vi "Diode-Test2-Array.vi"() -> ()   [LabVIEW 2020]
uses:
  Diode-SCPI-Driver/Diode-Keyword.ctl
panel:
  in  "Stop":bool
  out "Waveform Graph":u16[][](graph)=[[6664, 5392, 4415, 3740, 3338, 2832, 2456, 2200, 1952, 1855, 1920, 1848, 1808, 1698, 1703, 1756, 1820, 1796, 1664, 1584, 1495, 1648, 1584, 1536, 1416, 1424, 1432, 1468, 1588, 1552, 1480, 1488, 1536, 1388, 1432, 1468, 1592, 1576, 1465, 1590, 1580, 1584, 1488, 1536, 1384, 1408, 1343, 1467, 1594, 1584, 1552, 1456, 1492, 1544, 1464, 1536, 1416, 1418, 1469, 1576, 1488, 1540, 1424, 1462, 1542, 1538, 1420, 1470, 1597, 1599, 1672, 1591, 1599, 1696, 1599, 1680, 1664, 1544, 1468, 1557, 1521, 1550, 1560, 1468, 1595, 1592, 1568, 1458, 1577, 1510, 1595, 1627, 1664, 1569, 1432, 1498, 1592, 1570, 1536, 1386, 1407, 1570, 1536, 1410, 1408, 1408, 1340, 1424, 1425, 1416, 1409, 1408, 1343, 1462, 1599, 1664, 1577, 1484, 1564, 1534, 1720, 1744, 1727, 1855, 1855, 1936, 1820, 1836, 1776, 1808, 1688, 1681, 1599, 1705, 1672, 1596, 1599, 1680, 1664, 1550, 1570, 1468, 1597, 1592, 1554, 1518, 1664, 1558, 1587, 1564, 1552, 1460, 1552, 1460, 1536, 1424, 1416, 1424, 1414, 1471, 1664, 1561, 1496, 1593, 1560, 1496, 1568, 1464, 1558, 1536, 1430, 1492, 1590, 1564, 1568, 1432, 1488, 1544, 1457, 1470, 1632, 1537, 1424, 1424, 1424, 1456, 1458, 1588, 1536, 1426, 1456, 1471, 1664, 1560, 1492, 1553, 1458, 1577, 1470, 1656, 1672, 1592, 1578, 1548, 1536, 1343, 1456, 1498, 1594, 1598, 1664, 1578, 1562, 1567, 1599, 1668, 1595, 1632, 1536, 1408, 1342, 1490, 1552, 1456, 1490, 1576, 1470, 1664, 1584, 1504, 1514, 1599, 1668, 1599, 1680, 1598, 1680, 1599, 1688, 1688, 1688, 1680, 1632, 1560, 1496, 1546, 1536, 1408, 1342, 1470, 1632, 1552, 1456, 1494, 1599, 1599, 1680, 1664, 1577, 1496, 1584, 1536, 1343, 1492, 1560, 1494, 1592, 1579, 1552, 1454, 1560, 1536, 1343, 1492, 1560, 1504, 1514, 1593, 1570, 1552, 1432, 1468, 1580, 1552, 1454, 1560, 1538, 1436, 1552, 1424, 1443, 1456, 1536, 1342, 1491, 1552, 1447, 1520, 1598, 1599, 1698, 1688, 1690, 1720, 1776, 1724, 1794, 1672, 1680, 1598, 1670, 1672, 1666, 1592, 1595, 1580, 1584, 1468, 1594, 1598, 1664, 1566, 1584, 1538, 1457, 1492, 1584, 1497, 1584, 1496, 1598, 1664, 1560, 1556, 1468, 1592, 1560, 1536, 1408, 1336, 1380, 1333, 1392, 1343, 1499, 1596, 1664, 1552, 1474, 1496, 1571, 1496, 1579, 1544, 1449, 1468, 1580, 1536, 1418, 1456, 1536, 1408, 1343, 1470, 1599, 1672, 1594, 1648, 1584, 1544, 1422, 1536, 1392, 1426, 1466, 1588, 1546, 1279, 1598, 1680, 1664, 1568, 1465, 1500, 1664, 1552, 1462, 1592, 1570, 1471, 1664, 1552, 1471, 1597, 1636, 1540, 1488, 1536, 1410, 1416, 1456, 1464, 1536, 1416, 1408, 1343, 1497, 1568, 1456, 1504, 1536, 1408, 1336, 1343, 1470, 1599, 1664, 1584, 1439, 1599, 1672, 1599, 1670, 1686, 1727, 1851, 1822, 1853, 1842, 1792, 1664, 1554, 1552, 1436, 1552, 1464, 1544, 1424, 1433, 1470, 1596, 1599, 1680, 1664, 1560, 1491, 1580, 1560, 1468, 1599, 1664, 1578, 1518, 1696, 1596, 1621, 1576, 1538, 1432, 1536, 1340, 1464, 1544, 1440, 1479, 1577, 1470, 1664, 1588, 1569, 1448, 1464, 1568, 1420, 1475, 1496, 1634, 1538, 1490, 1548, 1536, 1343, 1488, 1536, 1410, 1408, 1408, 1340, 1416, 1416, 1433, 1468, 1587, 1558, 1576, 1490, 1592, 1556, 1467, 1571, 1536, 1424, 1408, 1408, 1311, 1442, 1468, 1570, 1536, 1416, 1412, 1441, 1416, 1432, 1439, 1596, 1598, 1648, 1599, 1672, 1632, 1524, 1706, 1678, 1748, 1724, 1814, 1749, 1792, 1590, 1664, 1560, 1536, 1408, 1394, 1424, 1456, 1460, 1536, 1408, 1343, 1463, 1567, 1598, 1672, 1599, 1680, 1598, 1680, 1599, 1672, 1599, 1696, 1598, 1681, 1664, 1576, 1508, 1552, 1464, 1536, 1408, 1340, 1430, 1470, 1667, 1599, 1700, 1664, 1589, 1552, 1459, 1520, 1582, 1584, 1550, 1500, 1664, 1536, 1424, 1428, 1536, 1340, 1408, 1343, 1459, 1538, 1461, 1516, 1599, 1680, 1598, 1676, 1712, 1684, 1692, 1736, 1705, 1676, 1696, 1664, 1554, 1506, 1598, 1622, 1680, 1599, 1680, 1596, 1599, 1672, 1590, 1596, 1599, 1672, 1664, 1569, 1464, 1536, 1416, 1408, 1393, 1408, 1343, 1464, 1560, 1470, 1665, 1576, 1536, 1408, 1337, 1343, 1432, 1507, 1552, 1475, 1471, 1636, 1596, 1599, 1664, 1590, 1594, 1618, 1576, 1554, 1464, 1554, 1492, 1568, 1468, 1568, 1450, 1552, 1428, 1471, 1664, 1559, 1548, 1471, 1664, 1560, 1536, 1343, 1536, 1341, 1425, 1424, 1442, 1436, 1550, 1520, 1590, 1594, 1664, 1552, 1470, 1598, 1684, 1664, 1592, 1536, 1426, 1464, 1538, 1436, 1568, 1420, 1490, 1548, 1506, 1552, 1463, 1568, 1470, 1599, 1664, 1574, 1568, 1536, 1408, 1343, 1466, 1566, 1599, 1664, 1585, 1512, 1584, 1508, 1568, 1465, 1536, 1424, 1412, 1441, 1408, 1343, 1458, 1552, 1450, 1536, 1416, 1424, 1410, 1448, 1468, 1584, 1510, 1597, 1599, 1648, 1594, 1599, 1672, 1599, 1670, 1696, 1664, 1560, 1506, 1570, 1495, 1599, 1680, 1664, 1542, 1536, 1392, 1408, 1408, 1342, 1471, 1598, 1676, 1670, 1664, 1596, 1584, 1538, 1424, 1476, 1468, 1596, 1564, 1566, 1576, 1536, 1343, 1494, 1598, 1682, 1672, 1631, 1688, 1680, 1597, 1634, 1592, 1555, 1536, 1394, 1432, 1494, 1582, 1664, 1536, 1450, 1492, 1574, 1503, 1684, 1694, 1812, 1704, 1715, 1727, 1851, 1840, 1760, 1692, 1739, 1727, 1854, 1896, 1840, 1758, 1855, 1886, 1953, 1852, 1855, 1900, 1855, 1823, 1855, 1920, 1840, 1726, 1848, 1798, 1753, 1663, 1816, 1727, 1840, 1776, 1751, 1840, 1808, 1698, 1692, 1738, 1725, 1824, 1668, 1664, 1548, 1536, 1343, 1470, 1624, 1599, 1664, 1584, 1536, 1408, 1342, 1459, 1536, 1408, 1343, 1470, 1598, 1680, 1664, 1566, 1598, 1672, 1590, 1599, 1664, 1586, 1552, 1464, 1548, 1465, 1574, 1552, 1455, 1564, 1568, 1432, 1536, 1332, 1408, 1326, 1432, 1454, 1596, 1576, 1538, 1432, 1470, 1630, 1680, 1640, 1594, 1588, 1598, 1664, 1584, 1536, 1401, 1444, 1456, 1504, 1488, 1542, 1460, 1560, 1470, 1666, 1598, 1680, 1628, 1599, 1674, 1696, 1599, 1664, 1586, 1584, 1503, 1689, 1684, 1672, 1634, 1592, 1570, 1488, 1552, 1436, 1538, 1424, 1440, 1432, 1471, 1664, 1584, 1500, 1595, 1594, 1599, 1700, 1664, 1578, 1560, 1536, 1342, 1488, 1486, 1624, 1566, 1599, 1599, 1694, 1723, 1842, 1792, 1599, 1688, 1704, 1668, 1639, 1664, 1584, 1504, 1536, 1408, 1342, 1460, 1592, 1576, 1471, 1664, 1565, 1544, 1440, 1456, 1457, 1520, 1552, 1470, 2860, 2489, 2304, 1855, 1928, 1850, 1855, 1952, 1846, 1872, 574, 831, 1036, 1059, 1048, 1074, 1087, 1210, 1343, 1440, 1440, 1460, 1552, 1440, 1456]]
  out "array":u16[][](array[numeric])=[[6664, 5392, 4415, 3740, 3338, 2832, 2456, 2200, 1952, 1855, 1920, 1848, 1808, 1698, 1703, 1756, 1820, 1796, 1664, 1584, 1495, 1648, 1584, 1536, 1416, 1424, 1432, 1468, 1588, 1552, 1480, 1488, 1536, 1388, 1432, 1468, 1592, 1576, 1465, 1590, 1580, 1584, 1488, 1536, 1384, 1408, 1343, 1467, 1594, 1584, 1552, 1456, 1492, 1544, 1464, 1536, 1416, 1418, 1469, 1576, 1488, 1540, 1424, 1462, 1542, 1538, 1420, 1470, 1597, 1599, 1672, 1591, 1599, 1696, 1599, 1680, 1664, 1544, 1468, 1557, 1521, 1550, 1560, 1468, 1595, 1592, 1568, 1458, 1577, 1510, 1595, 1627, 1664, 1569, 1432, 1498, 1592, 1570, 1536, 1386, 1407, 1570, 1536, 1410, 1408, 1408, 1340, 1424, 1425, 1416, 1409, 1408, 1343, 1462, 1599, 1664, 1577, 1484, 1564, 1534, 1720, 1744, 1727, 1855, 1855, 1936, 1820, 1836, 1776, 1808, 1688, 1681, 1599, 1705, 1672, 1596, 1599, 1680, 1664, 1550, 1570, 1468, 1597, 1592, 1554, 1518, 1664, 1558, 1587, 1564, 1552, 1460, 1552, 1460, 1536, 1424, 1416, 1424, 1414, 1471, 1664, 1561, 1496, 1593, 1560, 1496, 1568, 1464, 1558, 1536, 1430, 1492, 1590, 1564, 1568, 1432, 1488, 1544, 1457, 1470, 1632, 1537, 1424, 1424, 1424, 1456, 1458, 1588, 1536, 1426, 1456, 1471, 1664, 1560, 1492, 1553, 1458, 1577, 1470, 1656, 1672, 1592, 1578, 1548, 1536, 1343, 1456, 1498, 1594, 1598, 1664, 1578, 1562, 1567, 1599, 1668, 1595, 1632, 1536, 1408, 1342, 1490, 1552, 1456, 1490, 1576, 1470, 1664, 1584, 1504, 1514, 1599, 1668, 1599, 1680, 1598, 1680, 1599, 1688, 1688, 1688, 1680, 1632, 1560, 1496, 1546, 1536, 1408, 1342, 1470, 1632, 1552, 1456, 1494, 1599, 1599, 1680, 1664, 1577, 1496, 1584, 1536, 1343, 1492, 1560, 1494, 1592, 1579, 1552, 1454, 1560, 1536, 1343, 1492, 1560, 1504, 1514, 1593, 1570, 1552, 1432, 1468, 1580, 1552, 1454, 1560, 1538, 1436, 1552, 1424, 1443, 1456, 1536, 1342, 1491, 1552, 1447, 1520, 1598, 1599, 1698, 1688, 1690, 1720, 1776, 1724, 1794, 1672, 1680, 1598, 1670, 1672, 1666, 1592, 1595, 1580, 1584, 1468, 1594, 1598, 1664, 1566, 1584, 1538, 1457, 1492, 1584, 1497, 1584, 1496, 1598, 1664, 1560, 1556, 1468, 1592, 1560, 1536, 1408, 1336, 1380, 1333, 1392, 1343, 1499, 1596, 1664, 1552, 1474, 1496, 1571, 1496, 1579, 1544, 1449, 1468, 1580, 1536, 1418, 1456, 1536, 1408, 1343, 1470, 1599, 1672, 1594, 1648, 1584, 1544, 1422, 1536, 1392, 1426, 1466, 1588, 1546, 1279, 1598, 1680, 1664, 1568, 1465, 1500, 1664, 1552, 1462, 1592, 1570, 1471, 1664, 1552, 1471, 1597, 1636, 1540, 1488, 1536, 1410, 1416, 1456, 1464, 1536, 1416, 1408, 1343, 1497, 1568, 1456, 1504, 1536, 1408, 1336, 1343, 1470, 1599, 1664, 1584, 1439, 1599, 1672, 1599, 1670, 1686, 1727, 1851, 1822, 1853, 1842, 1792, 1664, 1554, 1552, 1436, 1552, 1464, 1544, 1424, 1433, 1470, 1596, 1599, 1680, 1664, 1560, 1491, 1580, 1560, 1468, 1599, 1664, 1578, 1518, 1696, 1596, 1621, 1576, 1538, 1432, 1536, 1340, 1464, 1544, 1440, 1479, 1577, 1470, 1664, 1588, 1569, 1448, 1464, 1568, 1420, 1475, 1496, 1634, 1538, 1490, 1548, 1536, 1343, 1488, 1536, 1410, 1408, 1408, 1340, 1416, 1416, 1433, 1468, 1587, 1558, 1576, 1490, 1592, 1556, 1467, 1571, 1536, 1424, 1408, 1408, 1311, 1442, 1468, 1570, 1536, 1416, 1412, 1441, 1416, 1432, 1439, 1596, 1598, 1648, 1599, 1672, 1632, 1524, 1706, 1678, 1748, 1724, 1814, 1749, 1792, 1590, 1664, 1560, 1536, 1408, 1394, 1424, 1456, 1460, 1536, 1408, 1343, 1463, 1567, 1598, 1672, 1599, 1680, 1598, 1680, 1599, 1672, 1599, 1696, 1598, 1681, 1664, 1576, 1508, 1552, 1464, 1536, 1408, 1340, 1430, 1470, 1667, 1599, 1700, 1664, 1589, 1552, 1459, 1520, 1582, 1584, 1550, 1500, 1664, 1536, 1424, 1428, 1536, 1340, 1408, 1343, 1459, 1538, 1461, 1516, 1599, 1680, 1598, 1676, 1712, 1684, 1692, 1736, 1705, 1676, 1696, 1664, 1554, 1506, 1598, 1622, 1680, 1599, 1680, 1596, 1599, 1672, 1590, 1596, 1599, 1672, 1664, 1569, 1464, 1536, 1416, 1408, 1393, 1408, 1343, 1464, 1560, 1470, 1665, 1576, 1536, 1408, 1337, 1343, 1432, 1507, 1552, 1475, 1471, 1636, 1596, 1599, 1664, 1590, 1594, 1618, 1576, 1554, 1464, 1554, 1492, 1568, 1468, 1568, 1450, 1552, 1428, 1471, 1664, 1559, 1548, 1471, 1664, 1560, 1536, 1343, 1536, 1341, 1425, 1424, 1442, 1436, 1550, 1520, 1590, 1594, 1664, 1552, 1470, 1598, 1684, 1664, 1592, 1536, 1426, 1464, 1538, 1436, 1568, 1420, 1490, 1548, 1506, 1552, 1463, 1568, 1470, 1599, 1664, 1574, 1568, 1536, 1408, 1343, 1466, 1566, 1599, 1664, 1585, 1512, 1584, 1508, 1568, 1465, 1536, 1424, 1412, 1441, 1408, 1343, 1458, 1552, 1450, 1536, 1416, 1424, 1410, 1448, 1468, 1584, 1510, 1597, 1599, 1648, 1594, 1599, 1672, 1599, 1670, 1696, 1664, 1560, 1506, 1570, 1495, 1599, 1680, 1664, 1542, 1536, 1392, 1408, 1408, 1342, 1471, 1598, 1676, 1670, 1664, 1596, 1584, 1538, 1424, 1476, 1468, 1596, 1564, 1566, 1576, 1536, 1343, 1494, 1598, 1682, 1672, 1631, 1688, 1680, 1597, 1634, 1592, 1555, 1536, 1394, 1432, 1494, 1582, 1664, 1536, 1450, 1492, 1574, 1503, 1684, 1694, 1812, 1704, 1715, 1727, 1851, 1840, 1760, 1692, 1739, 1727, 1854, 1896, 1840, 1758, 1855, 1886, 1953, 1852, 1855, 1900, 1855, 1823, 1855, 1920, 1840, 1726, 1848, 1798, 1753, 1663, 1816, 1727, 1840, 1776, 1751, 1840, 1808, 1698, 1692, 1738, 1725, 1824, 1668, 1664, 1548, 1536, 1343, 1470, 1624, 1599, 1664, 1584, 1536, 1408, 1342, 1459, 1536, 1408, 1343, 1470, 1598, 1680, 1664, 1566, 1598, 1672, 1590, 1599, 1664, 1586, 1552, 1464, 1548, 1465, 1574, 1552, 1455, 1564, 1568, 1432, 1536, 1332, 1408, 1326, 1432, 1454, 1596, 1576, 1538, 1432, 1470, 1630, 1680, 1640, 1594, 1588, 1598, 1664, 1584, 1536, 1401, 1444, 1456, 1504, 1488, 1542, 1460, 1560, 1470, 1666, 1598, 1680, 1628, 1599, 1674, 1696, 1599, 1664, 1586, 1584, 1503, 1689, 1684, 1672, 1634, 1592, 1570, 1488, 1552, 1436, 1538, 1424, 1440, 1432, 1471, 1664, 1584, 1500, 1595, 1594, 1599, 1700, 1664, 1578, 1560, 1536, 1342, 1488, 1486, 1624, 1566, 1599, 1599, 1694, 1723, 1842, 1792, 1599, 1688, 1704, 1668, 1639, 1664, 1584, 1504, 1536, 1408, 1342, 1460, 1592, 1576, 1471, 1664, 1565, 1544, 1440, 1456, 1457, 1520, 1552, 1470, 2860, 2489, 2304, 1855, 1928, 1850, 1855, 1952, 1846, 1872, 574, 831, 1036, 1059, 1048, 1074, 1087, 1210, 1343, 1440, 1440, 1460, 1552, 1440, 1456]]
  in  "max bytes to read (500)":i32=10000
  in  "Diode Keyword":T1={"Keyword"="DIOD:TRAC:YARR", "Gettable"=TRUE, "Settable"=FALSE, "Is Array"=FALSE, "Data Type"="string", "Description"="Identify the instrument."}
  out "Response":string="6664,5392,4415,3740,3338,2832,2456,2200,1952,1855,1920,1848,1808,1698,1703,1756,1820,1796,1664,1584,1495,1648,1584,1536,1416,1424,1432,1468,1588,1552,1480,1488,1536,1388,1432,1468,1592,1576,1465,1590,1580,1584,1488,1536,1384,1408,1343,1467,1594,1584,1552,1456,1492,1544,1464,1536,1416,1418,1469,1576,1488,1540,1424,1462,1542,1538,1420,1470,1597,1599,1672,1591,1599,1696,1599,1680,1664,1544,1468,1557,1521,1550,1560,1468,1595,1592,1568,1458,1577,1510,1595,1627,1664,1569,1432,1498,1592,1570,1536,1386,1407,1570,1536,1410,1408,1408,1340,1424,1425,1416,1409,1408,1343,1462,1599,1664,1577,1484,1564,1534,1720,1744,1727,1855,1855,1936,1820,1836,1776,1808,1688,1681,1599,1705,1672,1596,1599,1680,1664,1550,1570,1468,1597,1592,1554,1518,1664,1558,1587,1564,1552,1460,1552,1460,1536,1424,1416,1424,1414,1471,1664,1561,1496,1593,1560,1496,1568,1464,1558,1536,1430,1492,1590,1564,1568,1432,1488,1544,1457,1470,1632,1537,1424,1424,1424,1456,1458,1588,1536,1426,1456,1471,1664,1560,1492,1553,1458,1577,1470,1656,1672,1592,1578,1548,1536,1343,1456,1498,1594,1598,1664,1578,1562,1567,1599,1668,1595,1632,1536,1408,1342,1490,1552,1456,1490,1576,1470,1664,1584,1504,1514,1599,1668,1599,1680,1598,1680,1599,1688,1688,1688,1680,1632,1560,1496,1546,1536,1408,1342,1470,1632,1552,1456,1494,1599,1599,1680,1664,1577,1496,1584,1536,1343,1492,1560,1494,1592,1579,1552,1454,1560,1536,1343,1492,1560,1504,1514,1593,1570,1552,1432,1468,1580,1552,1454,1560,1538,1436,1552,1424,1443,1456,1536,1342,1491,1552,1447,1520,1598,1599,1698,1688,1690,1720,1776,1724,1794,1672,1680,1598,1670,1672,1666,1592,1595,1580,1584,1468,1594,1598,1664,1566,1584,1538,1457,1492,1584,1497,1584,1496,1598,1664,1560,1556,1468,1592,1560,1536,1408,1336,1380,1333,1392,1343,1499,1596,1664,1552,1474,1496,1571,1496,1579,1544,1449,1468,1580,1536,1418,1456,1536,1408,1343,1470,1599,1672,1594,1648,1584,1544,1422,1536,1392,1426,1466,1588,1546,1279,1598,1680,1664,1568,1465,1500,1664,1552,1462,1592,1570,1471,1664,1552,1471,1597,1636,1540,1488,1536,1410,1416,1456,1464,1536,1416,1408,1343,1497,1568,1456,1504,1536,1408,1336,1343,1470,1599,1664,1584,1439,1599,1672,1599,1670,1686,1727,1851,1822,1853,1842,1792,1664,1554,1552,1436,1552,1464,1544,1424,1433,1470,1596,1599,1680,1664,1560,1491,1580,1560,1468,1599,1664,1578,1518,1696,1596,1621,1576,1538,1432,1536,1340,1464,1544,1440,1479,1577,1470,1664,1588,1569,1448,1464,1568,1420,1475,1496,1634,1538,1490,1548,1536,1343,1488,1536,1410,1408,1408,1340,1416,1416,1433,1468,1587,1558,1576,1490,1592,1556,1467,1571,1536,1424,1408,1408,1311,1442,1468,1570,1536,1416,1412,1441,1416,1432,1439,1596,1598,1648,1599,1672,1632,1524,1706,1678,1748,1724,1814,1749,1792,1590,1664,1560,1536,1408,1394,1424,1456,1460,1536,1408,1343,1463,1567,1598,1672,1599,1680,1598,1680,1599,1672,1599,1696,1598,1681,1664,1576,1508,1552,1464,1536,1408,1340,1430,1470,1667,1599,1700,1664,1589,1552,1459,1520,1582,1584,1550,1500,1664,1536,1424,1428,1536,1340,1408,1343,1459,1538,1461,1516,1599,1680,1598,1676,1712,1684,1692,1736,1705,1676,1696,1664,1554,1506,1598,1622,1680,1599,1680,1596,1599,1672,1590,1596,1599,1672,1664,1569,1464,1536,1416,1408,1393,1408,1343,1464,1560,1470,1665,1576,1536,1408,1337,1343,1432,1507,1552,1475,1471,1636,1596,1599,1664,1590,1594,1618,1576,1554,1464,1554,1492,1568,1468,1568,1450,1552,1428,1471,1664,1559,1548,1471,1664,1560,1536,1343,1536,1341,1425,1424,1442,1436,1550,1520,1590,1594,1664,1552,1470,1598,1684,1664,1592,1536,1426,1464,1538,1436,1568,1420,1490,1548,1506,1552,1463,1568,1470,1599,1664,1574,1568,1536,1408,1343,1466,1566,1599,1664,1585,1512,1584,1508,1568,1465,1536,1424,1412,1441,1408,1343,1458,1552,1450,1536,1416,1424,1410,1448,1468,1584,1510,1597,1599,1648,1594,1599,1672,1599,1670,1696,1664,1560,1506,1570,1495,1599,1680,1664,1542,1536,1392,1408,1408,1342,1471,1598,1676,1670,1664,1596,1584,1538,1424,1476,1468,1596,1564,1566,1576,1536,1343,1494,1598,1682,1672,1631,1688,1680,1597,1634,1592,1555,1536,1394,1432,1494,1582,1664,1536,1450,1492,1574,1503,1684,1694,1812,1704,1715,1727,1851,1840,1760,1692,1739,1727,1854,1896,1840,1758,1855,1886,1953,1852,1855,1900,1855,1823,1855,1920,1840,1726,1848,1798,1753,1663,1816,1727,1840,1776,1751,1840,1808,1698,1692,1738,1725,1824,1668,1664,1548,1536,1343,1470,1624,1599,1664,1584,1536,1408,1342,1459,1536,1408,1343,1470,1598,1680,1664,1566,1598,1672,1590,1599,1664,1586,1552,1464,1548,1465,1574,1552,1455,1564,1568,1432,1536,1332,1408,1326,1432,1454,1596,1576,1538,1432,1470,1630,1680,1640,1594,1588,1598,1664,1584,1536,1401,1444,1456,1504,1488,1542,1460,1560,1470,1666,1598,1680,1628,1599,1674,1696,1599,1664,1586,1584,1503,1689,1684,1672,1634,1592,1570,1488,1552,1436,1538,1424,1440,1432,1471,1664,1584,1500,1595,1594,1599,1700,1664,1578,1560,1536,1342,1488,1486,1624,1566,1599,1599,1694,1723,1842,1792,1599,1688,1704,1668,1639,1664,1584,1504,1536,1408,1342,1460,1592,1576,1471,1664,1565,1544,1440,1456,1457,1520,1552,1470,2860,2489,2304,1855,1928,1850,1855,1952,1846,1872,574,831,1036,1059,1048,1074,1087,1210,1343,1440,1440,1460,1552,1440,1456\r\n"
  in  "IP Address of Device":string="192.168.203.151"
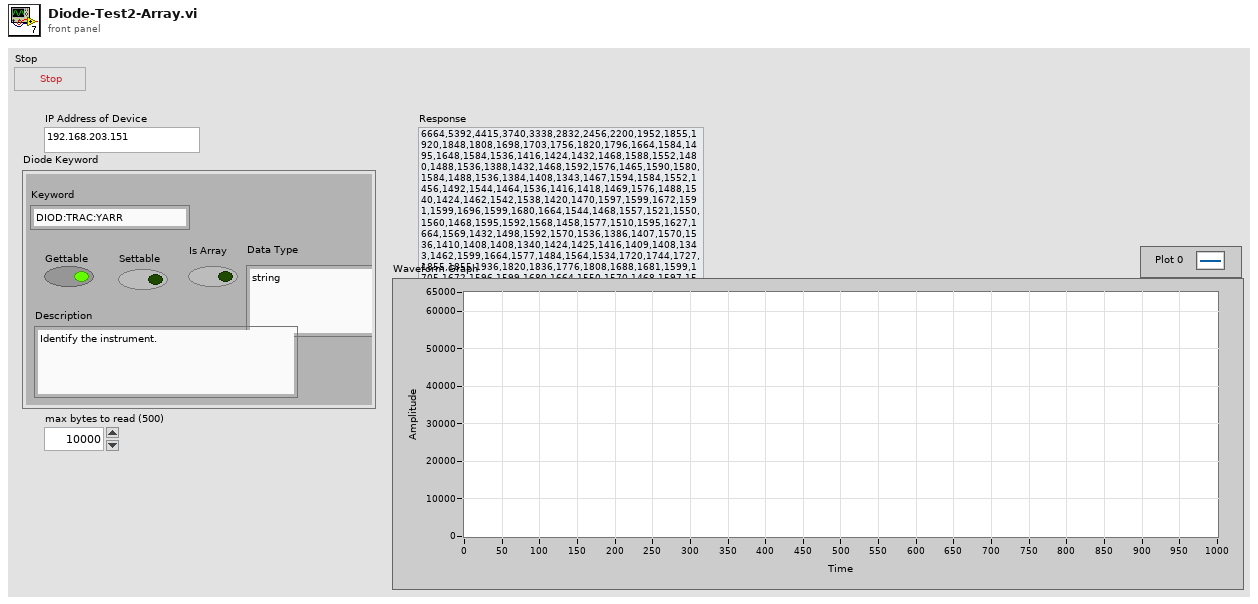
[diagram p1: front panel]
types:
  T1 = typedef "Diode-Keyword.ctl" = cluster{"Keyword":string, "Gettable":bool, "Settable":bool, "Is Array":bool, "Data Type":string, "Description":string}
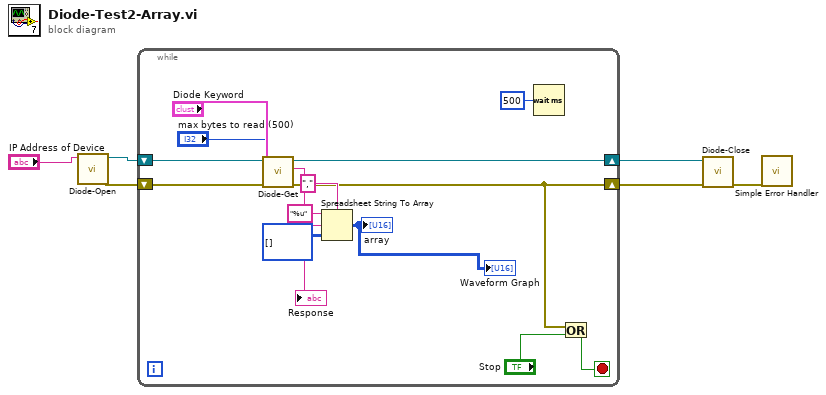
[diagram p0: block diagram]
diagram:
  n1 = call "Diode-Open.vi"("IP Address of Diode"="IP Address of Device") -> ("error out"=w1:errorcluster, "connection ID"=w4:refnum<k5>)  [unwired: 9 in]
  n2 = while {
    shift-right: [w18] -> w3
    shift-left: w4 -> [w19]
    shift-right: [w8] -> w2
    shift-left: w1 -> [w17]
    stop <- w7 stop-if-true
    n3 = call "Diode-Get.vi"("error in (no error)"=w17, "max bytes to read (10000)"="max bytes to read (500)", "Diode Keyword (leave off question mark)"="Diode Keyword", "connection ID"=w19) -> ("error out"=w8:errorcluster, "Response"=w15:string, "connection ID out"=w18:refnum<k5>)  [unwired: 4 in, 1 out]
    "Response" <- w15
    n4 = Spreadsheet String To Array(delimiter (Tab)=",", format string="%u", spreadsheet string=w15, array type (2D Dbl)=u16[][] []) -> (array=→"array" →"Waveform Graph":u16[][])
    n5 = Wait (ms)(milliseconds to wait=u32 500) -> ()  [unwired: 1 out]
    n6 = Or(x=w8, y="Stop") -> (x .or. y?=w7:bool)
  }
  n7 = call "Diode-Close.vi"("error in (no error)"=w2, "connection ID"=w3) -> ("error out"=w5:errorcluster)  [unwired: 9 in]
  n8 = call <vilib>:"Simple Error Handler.vi"("error in (no error)"=w5) -> ()  [unwired: 4 in, 5 out]
